vi "Read Meta Data (TCP Clst).vi"(6 "options":T3={"ignore timeout error"=TRUE, "timeout ms (1000)"=1000}, 8 "error in":errorcluster, 11 "connection info in":T1) -> (0 "error out":errorcluster, 1 "meta data":T2[](array[typedef]), 3 "connection info out":T1)   [LabVIEW 2013, in "NI STM.lvlib"]
doc: "This VI reads the meta data information from a remote computer. Use this VI to retrieve the variable names and types that a remote computer exports.\n\nThis VI parses the data and returns a cluster containing the meta data information."
uses:
  SubVIs/MetaDataElement.ctl
  TCP Read Options.ctl
  TCP Connection Info.ctl
  NI STM.lvlib
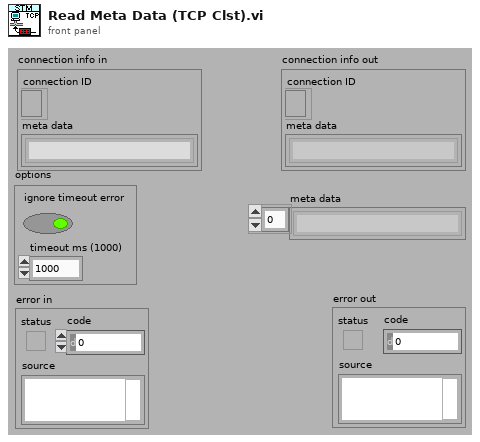
[diagram p1: front panel]
types:
  T1 = typedef "NI STM.lvlib/TCP Connection Info.ctl" = cluster{"connection ID":refnum<k5>, "meta data":T2[]}
  T2 = typedef "NI STM.lvlib/MetaDataElement.ctl" = string
  T3 = typedef "NI STM.lvlib/TCP Read Options.ctl" = cluster{"ignore timeout error":bool, "timeout ms (1000)":i32}
  T4 = enum16{"Standard", "Buffered", "CRLF", "Immediate"}
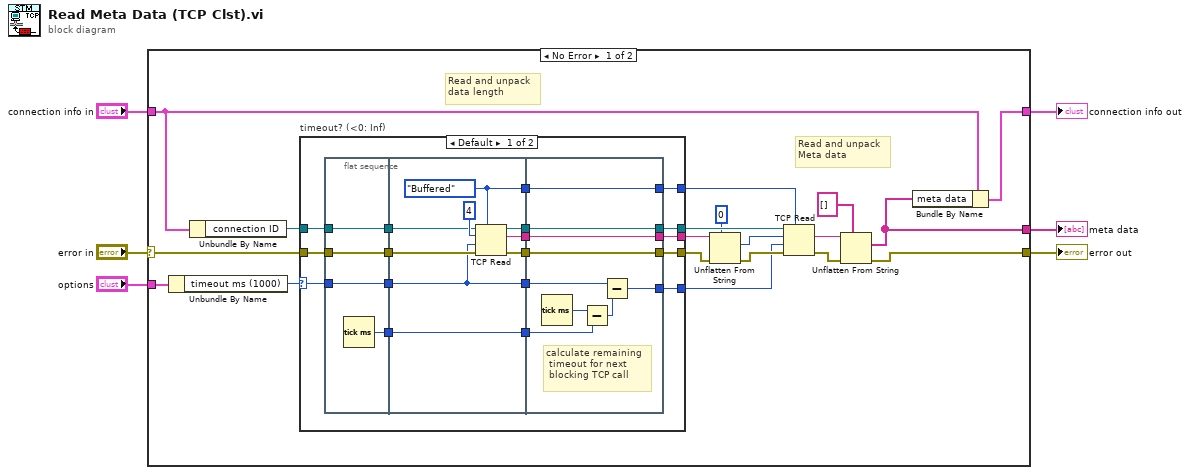
[diagram p0: block diagram]
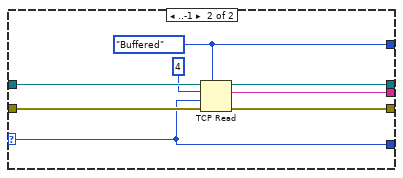
[diagram p2: hidden frame]
diagram:
  n1 = case shown="No Error" "error in" {
    selector: "error in" -> [w15 w75]
    tunnel: [w14 _] -> w6
    tunnel: [w25 w75] -> w5
    tunnel: [w13 w74] -> w1
    tunnel: "options" -> [w12 _]
    tunnel: "connection info in" -> [w10 w74]
    frame No Error {
      # "Read and unpack\nMeta data"
      # "Read and unpack\ndata length"
      n2 = Unbundle By Name(w12) -> ("timeout ms (1000)"=w8:i32)
      n3 = Unbundle By Name(w10) -> ("connection ID"=w11:refnum<k5>)
      n4 = case "timeout? (<0: Inf)" shown="Default" w8 {
        selector: w8 -> [w28 w67]
        tunnel: [w34 w73] -> w23
        tunnel: [w33 w72] -> w20
        tunnel: [w32 w71] -> w16
        tunnel: w15 -> [w31 w70]
        tunnel: w11 -> [w30 w69]
        tunnel: [w29 w67] -> w9
        tunnel: [w26 w66] -> w7
        frame Default {
          n5 = flat-sequence {
            tunnel: w28 -> [w45]
            tunnel: w30 -> [w46]
            tunnel: w31 -> [w47]
            tunnel: [w47] -> w43
            tunnel: [w46] -> w42
            tunnel: [w45] -> w41
            tunnel: [w44] -> w40
            tunnel: [w55] -> w39
            tunnel: [w54] -> w38
            tunnel: [w53] -> w37
            tunnel: w43 -> [w52]
            tunnel: w42 -> [w51]
            tunnel: w41 -> [w49]
            tunnel: w40 -> [w50]
            tunnel: [w50] -> w36
            tunnel: [w49] -> w35
            tunnel: [w48] -> w27
            tunnel: [w63] -> w32
            tunnel: [w64] -> w33
            tunnel: [w65] -> w34
            tunnel: w39 -> [w65]
            tunnel: w38 -> [w64]
            tunnel: w37 -> [w63]
            tunnel: w36 -> [w61]
            tunnel: w35 -> [w60]
            tunnel: [w58] -> w29
            tunnel: w27 -> [w57]
            tunnel: [w57] -> w26
            frame #0 {
              n6 = Tick Count (ms)() -> (millisecond timer value=w44:u32)
            }
            frame #1 {
              w48 = T4."Buffered" ("mode (standard)")
              n7 = TCP Read(connection ID=w51, bytes to read=4, error in (no error)=w52, 7:w48, 9:w49) -> (connection ID out=w55:refnum<k5>, data out=w54:string, error out=w53:errorcluster)
            }
            frame #2 {
              # "calculate remaining\n timeout for next\n blocking TCP call"
              n8 = Tick Count (ms)() -> (millisecond timer value=w62:u32)
              n9 = Subtract(x=w62, y=w61) -> (x-y=w59:u32)
              n10 = Subtract(x=w60, y=w59) -> (x-y=w58:u32)
            }
          }
        }
        frame ..-1 {
          w66 = T4."Buffered" ("mode (standard)")
          n11 = TCP Read(connection ID=w69, bytes to read=4, error in (no error)=w70, 7:w66, 9:w67) -> (connection ID out=w73:refnum<k5>, data out=w72:string, error out=w71:errorcluster)
        }
      }
      n12 = Unflatten From String(type=0 ("bytes to read"), binary string=w20, error in (no error)=w16) -> (value=w17:i32, error out=w18:errorcluster)  [unwired: 3 out]
      n13 = TCP Read(connection ID=w23, bytes to read=w17, error in (no error)=w18, 7:w7, 9:w9) -> (data out=w22:string, error out=w21:errorcluster)  [unwired: 1 out]
      n14 = Unflatten From String(type=T2[] [] ("Meta data"), binary string=w22, error in (no error)=w21) -> (value=w14:T2[], error out=w25:errorcluster)  [unwired: 3 out]
      n15 = Bundle By Name(cluster=w10, "meta data"=w14) -> (w13:T1)
    }
    frame Error {
    }
  }
  "meta data" <- w6
  "error out" <- w5
  "connection info out" <- w1
